vi "detElementNameNoAttributes.vi"(8 "error in (no error)":errorcluster, 10 "XML In":string, 11 "ReadElement Out":refnum<class "XMLParser.lvclass">) -> (0 "error out":errorcluster, 2 "ElementName":string, 3 "ReadElement Out":refnum<class "XMLParser.lvclass">)   [LabVIEW 2014, in "XML.lvlib" / "XMLParser.lvclass"]
doc: "This mehtod determines the element name if the are no attributes detected. This method will fail if there are attributes in the XML."
uses:
  <userlib>/Common/XML/XMLParser/XMLParser.lvclass
  <userlib>/Common/XML/XMLParser/XMLParser.lvclass/XMLParser.ctl
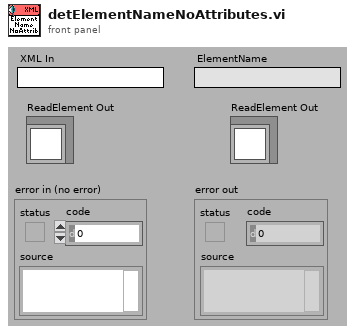
[diagram p1: front panel]
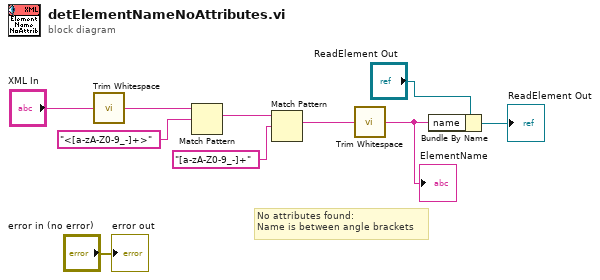
[diagram p0: block diagram]
diagram:
  # "No attributes found:\nName is between angle brackets"
  n1 = call <vilib>:"Trim Whitespace.vi"("string"="XML In") -> ("trimmed string"=w7:string)  [unwired: 1 in]
  n2 = Match Pattern(string=w7, regular expression="<[a-zA-Z0-9_-]+>") -> (match substring=w9:string)  [unwired: 1 in, 3 out]
  n3 = Match Pattern(string=w9, regular expression="[a-zA-Z0-9_-]+") -> (match substring=w3:string)  [unwired: 1 in, 3 out]
  n4 = call <vilib>:"Trim Whitespace.vi"("string"=w3) -> ("trimmed string"=w2:string)  [unwired: 1 in]
  "ElementName" <- w2
  n5 = Bundle By Name(cluster="ReadElement Out", "name"=w2) -> (→"ReadElement Out":refnum<class "XMLParser.lvclass">)
  "error out" <- "error in (no error)"
